vi "Periodic Tasks.vi"(8 "error in":errorcluster) -> ()   [LabVIEW 2016]
doc: "This VI runs in parallel to other tasks. It can contain as many user-defined periodic loops as you need. These can carry out PID or other sorts of timed response."
uses:
  <vilib>/Rock Robotics/WPI/DriverStation/WPI_DriverStationRobotMode2.ctl
  <vilib>/Rock Robotics/Network Tables/NT Write Number.vi
  Robot Global Data.vi
  <vilib>/Rock Robotics/Network Tables/NT Write Boolean.vi
  <vilib>/Rock Robotics/Network Tables/NT Read String.vi
  <vilib>/Rock Robotics/Network Tables/NT Write String.vi
  <vilib>/Rock Robotics/Network Tables/NT Read Number.vi
  <vilib>/Rock Robotics/WPI/Utilities/WPI_GetSetVariantRefNum.vi
  <vilib>/Rock Robotics/Network Tables/NT Read Boolean.vi
  <vilib>/Rock Robotics/Network Tables/NT Write Numeric Array.vi
  <vilib>/Rock Robotics/Network Tables/NT Read Numeric Array.vi
panel:
  out "Shooter Speed":dbl=-0.0
  out "Shooter Encoder 2":dbl(graph)
  out "Shooter Encoder":dbl(graph)
  in  "Voltage Correction Factor":dbl=0.9725 format="%#_13g"
  in  "Ball Detection Fast Time (ms)":u32=20
  out "Channel 1 (Climb Motor)":dbl(graph)
  out "Channel 0 (Climb Motor)":dbl(graph)
  in  "Range":dbl=100.0 format="%#_13g"
  out "Averaged Values":dbl(graph)=25.833333333333332
  out "<5?":i16(graph)=1
  out "Image Width":dbl(graph)=26.0
  in  "Past array Width":dbl[](array[numeric])=[26.0, 26.0, 26.0, 25.0, 26.0, 26.0]
  out "Gear Orient":bool
  out "Gear In":bool
  out "1 Width":dbl=17.0
  out "1 X Axis":dbl=26.0
  out "2 Width":dbl=8.5
  out "2 X Axis":dbl=13.0
  in  "Past array":dbl[](array[numeric])=[-10.0, -10.0, -10.0]
  in  "Lcal Pixy Out":dbl=-10.0
  # "Pixy Code V1 Variables\n      Only here for legacy support if V2 fails.\n\nPixy Code V2 varables are located in\n      \"Pixy Logic Core.vi\""
  # "Factor is 0.9725\nFor voltage 12.8"
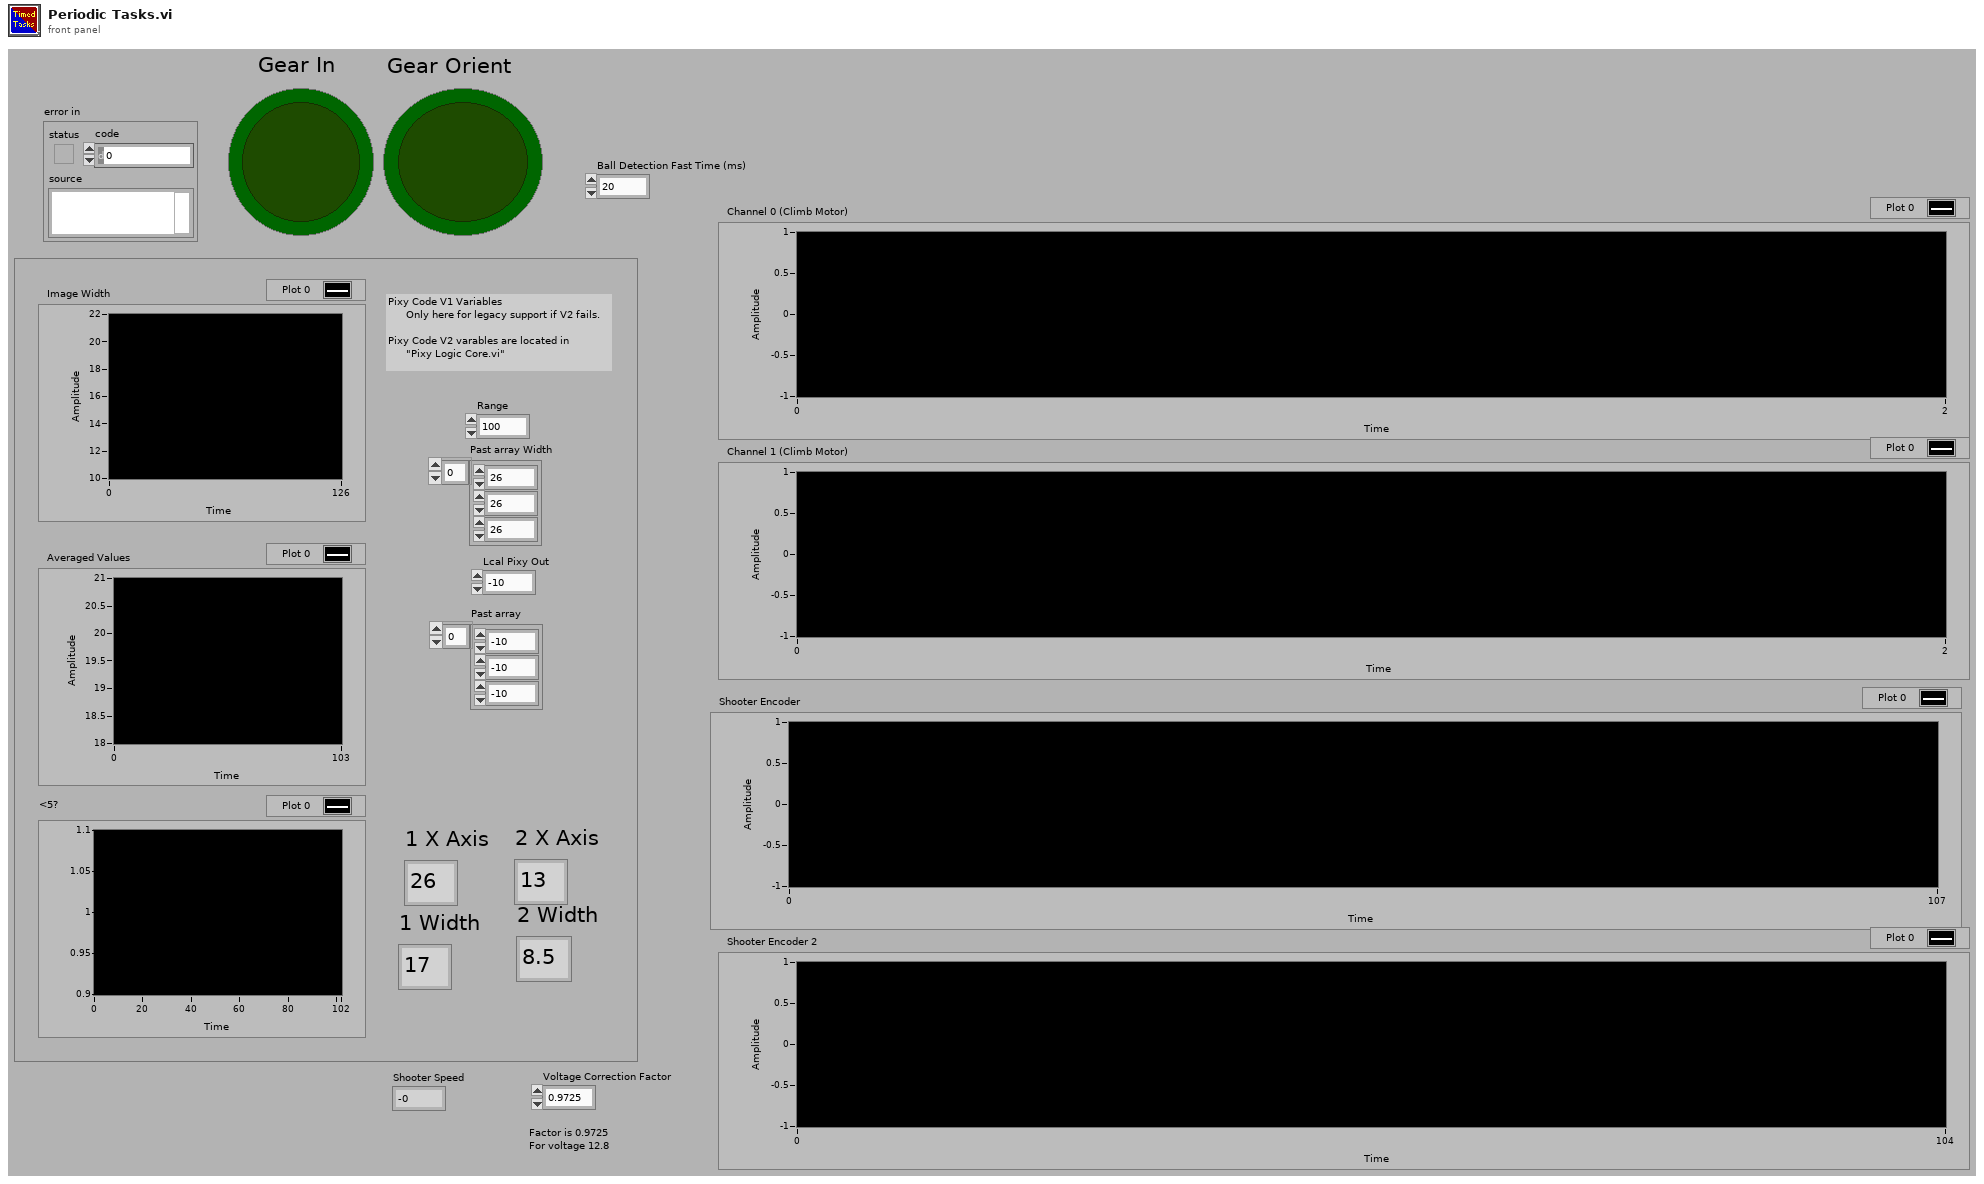
[diagram p1: front panel]
types:
  T1 = typedef "WPI_EncoderDevRef.ctl" = cluster{"DevStatus":errorcluster, "EncoderIndex":T2, "CounterIndex":T3, "DistancePerCount":dbl, "Decoding Type":T4}
  T2 = typedef "FPGA_EncoderIdx.ctl" = enum8{"Enc 0", "Enc 1", "Enc 2", "Enc 3", "Enc 4", "Enc 5", "Enc 6", "Enc 7", "Invalid"}
  T3 = typedef "FPGA_CounterCtrSystemIndex.ctl" = enum8{"Ctr 0", "Ctr 1", "Ctr 2", "Ctr 3", "Ctr 4", "Ctr 5", "Ctr 6", "Ctr 7", "Invalid"}
  T4 = typedef "WPI_EncoderType.ctl" = enum16{"1x", "2x", "4x"}
  T5 = typedef "WPI_SwitchDevRef.ctl" = cluster{"DevStatus":errorcluster, "DIO Channel":T6, "CntIndex":T3, "Normally Closed":bool}
  T6 = typedef "FPGA_DIOChannel.ctl" = enum8{"DIO 0", "DIO 1", "DIO 2", "DIO 3", "DIO 4", "DIO 5", "DIO 6", "DIO 7", "DIO 8", "DIO 9", "DIO MXP 0", "DIO MXP 1", "DIO MXP 2", "DIO MXP 3", "DIO MXP 4", "DIO MXP 5", "DIO MXP 6", "DIO MXP 7", "DIO MXP 8", "DIO MXP 9", "DIO MXP 10", "DIO MXP 11", "DIO MXP 12", "DIO MXP 13", "DIO MXP 14", "DIO MXP 15", "SPI Port CS1", "SPI Port CS2", "SPI Port CS3", "SPI Port MISO", "SPI Port MOSI", "Invalid"}
  T7 = typedef "WPI_ServoDeviceRef.ctl" = cluster{"DeviceStatus":errorcluster, "PWM Channel":T8, "DeadBand":T9}
  T8 = typedef "FPGA_DIOPWMChannel.ctl" = enum8{"PWM 0", "PWM 1", "PWM 2", "PWM 3", "PWM 4", "PWM 5", "PWM 6", "PWM 7", "PWM 8", "PWM 9", "PWM MXP 0", "PWM MXP 1", "PWM MXP 2", "PWM MXP 3", "PWM MXP 4", "PWM MXP 5", "PWM MXP 6", "PWM MXP 7", "PWM MXP 8", "PWM MXP 9", "Invalid"}
  T9 = typedef "WPI_PWMDeadband.ctl" = cluster{"Name":string, "maxPositivePwm":i32, "minPositivePwm":i32, "centerPwm":i32, "maxNegativePwm":i32, "minNegativePwm":i32, "angularRange":u16}
  T10 = typedef "WPI_JoystickDevRef.ctl" = cluster{"Device":T11}
  T11 = typedef "WPI_JoystickDeviceEnum.ctl" = enum16{"USB 0", "USB 1", "USB 2", "USB 3", "USB 4", "USB 5"}
  T12 = typedef "WPI_DriverStationRobotMode2.ctl" = enum16{"Autonomous Disabled", "Autonomous Enabled", "Teleop Disabled", "Teleop Enabled", "Disconnected", "Finish", "Test Disabled", "Test Enabled", "Emergency Stopped"}
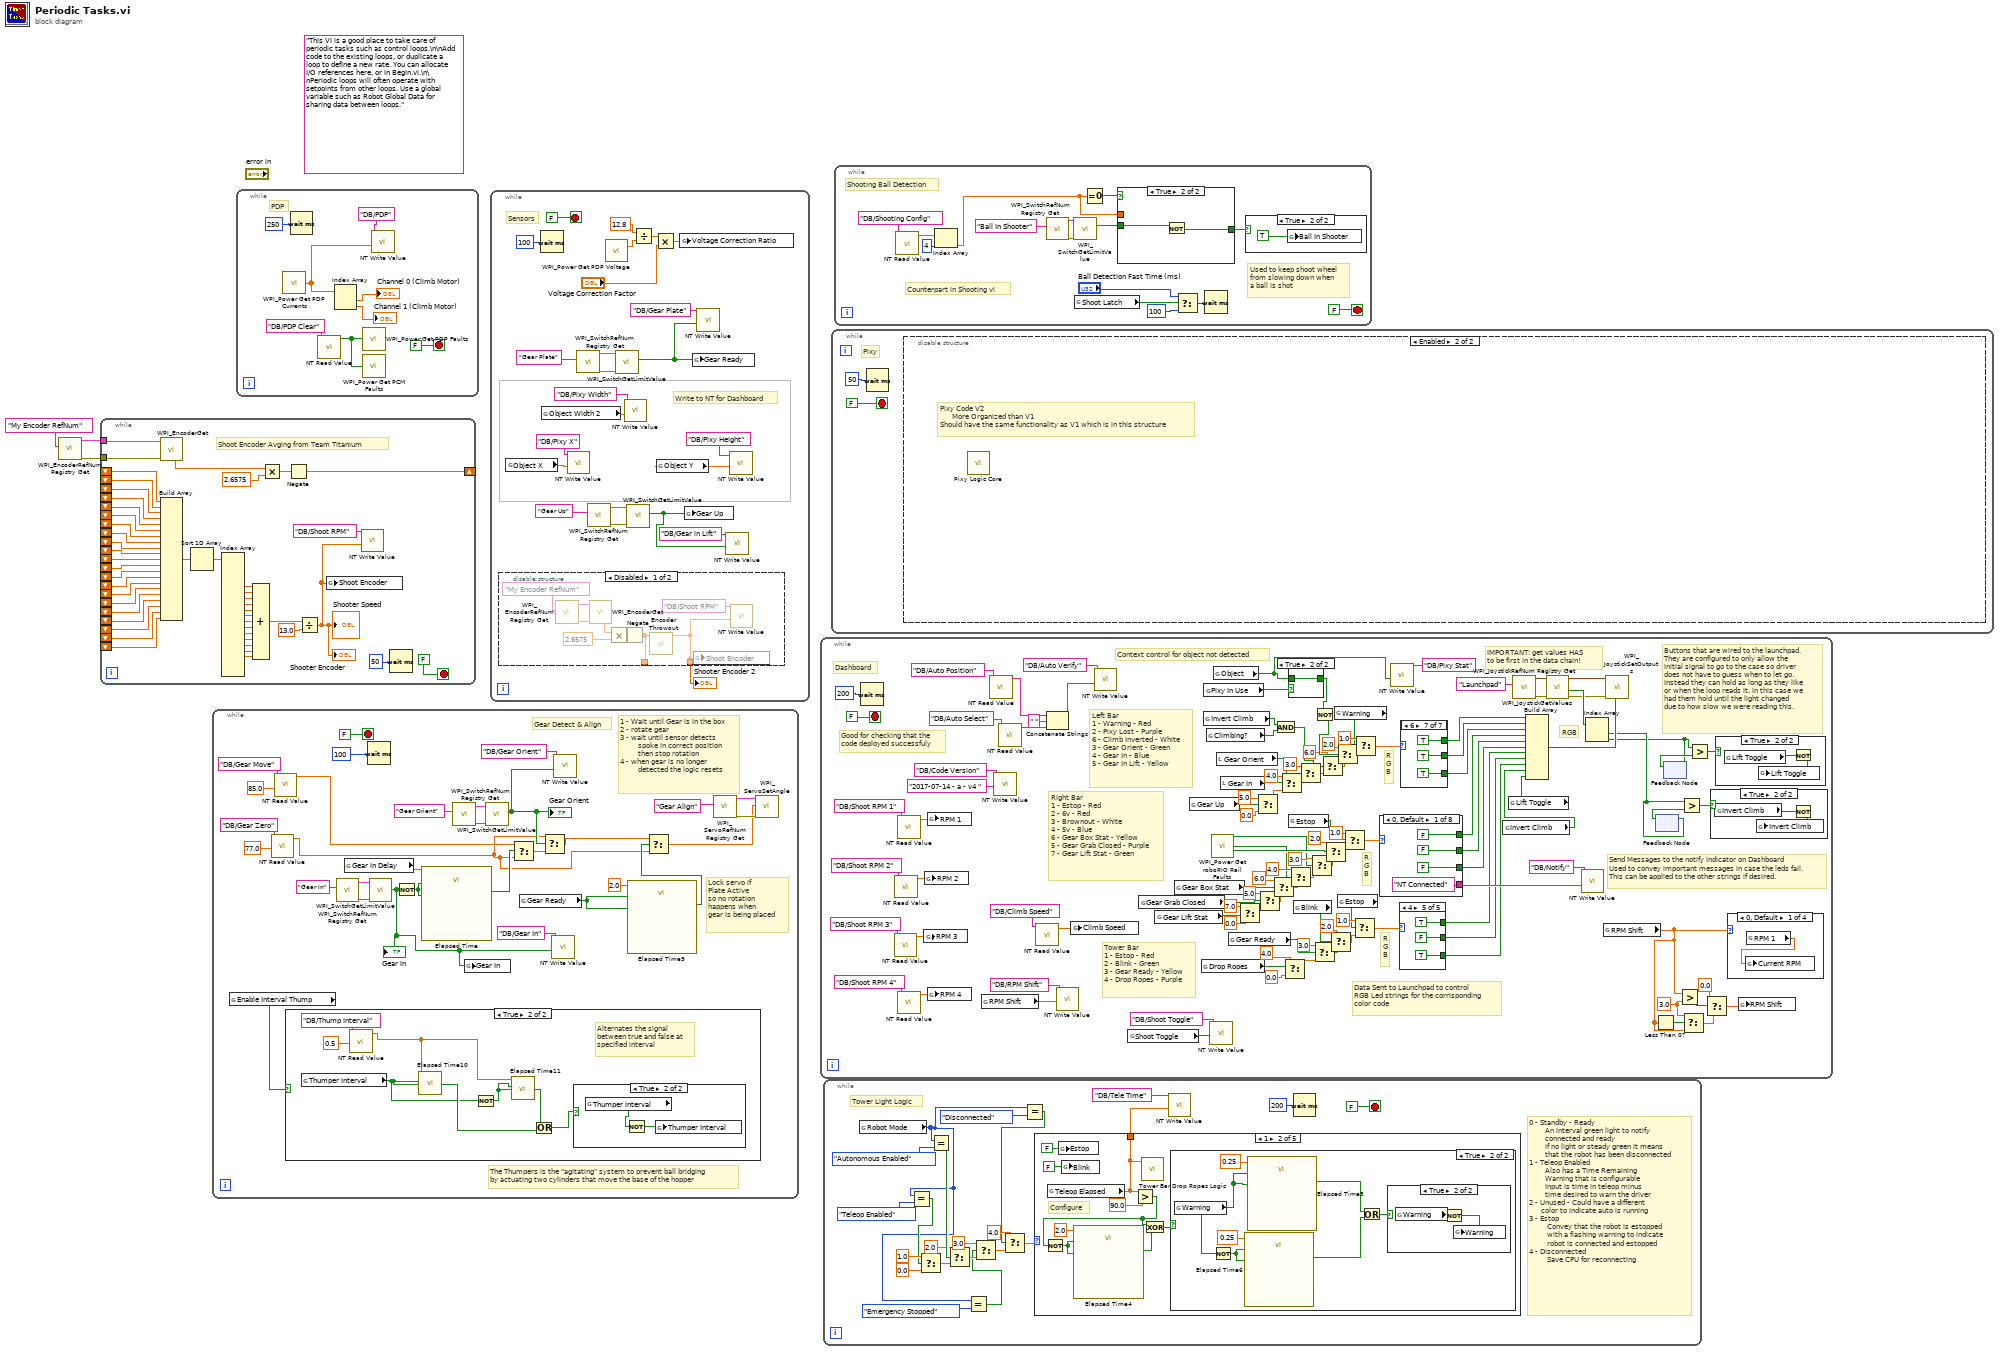
[diagram p0: block diagram]
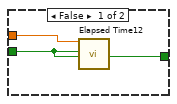
[diagram p2: hidden frame]
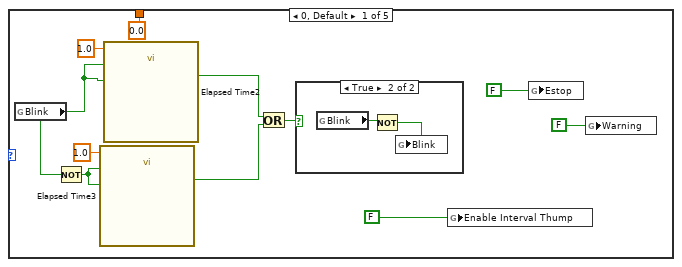
[diagram p4: hidden frame]
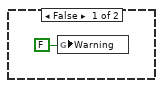
[diagram p6: hidden frame]
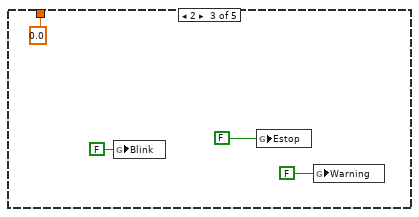
[diagram p8: hidden frame]
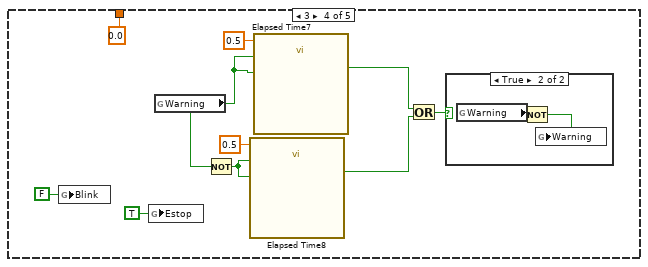
[diagram p9: hidden frame]
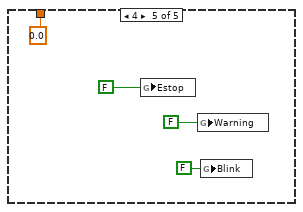
[diagram p11: hidden frame]
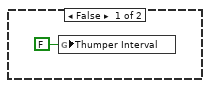
[diagram p12: hidden frame]
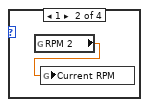
[diagram p14: hidden frame]
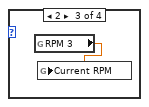
[diagram p15: hidden frame]
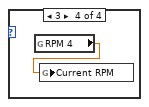
[diagram p16: hidden frame]
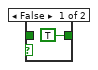
[diagram p19: hidden frame]
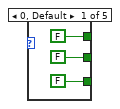
[diagram p20: hidden frame]
diagram:
  (unwired) "This VI is a good place to take care of periodic tasks such as control loops.\n\nAdd code to the existing loops, or duplicate a loop to define a new rate. You can allocate I/O references here, or in Begin.vi.\n\nPeriodic loops will often operate with setpoints from other loops. Use a global variable such as Robot Global Data for sharing data between loops."
  n1 = call <vilib>:"WPI_EncoderRefNum Registry Get.vi"("refnum name"="My Encoder RefNum") -> ("error out"=w1:errorcluster, "EncoderDevRef"=w2:T1)  [unwired: 9 in]
  n2 = while {
    tunnel: w2 -> [w49]
    shift-right: [w46] -> _
    shift-left: _ -> [w45]
    shift-left: _ -> [w44]
    shift-left: _ -> [w43]
    shift-left: _ -> [w42]
    shift-left: _ -> [w41]
    shift-left: _ -> [w40]
    shift-left: _ -> [w39]
    shift-left: _ -> [w38]
    shift-left: _ -> [w37]
    shift-left: _ -> [w36]
    shift-left: _ -> [w35]
    shift-left: _ -> [w34]
    shift-left: _ -> [w33]
    shift-left: _ -> [w32]
    shift-left: _ -> [w31]
    shift-left: _ -> [w30]
    shift-left: _ -> [w17]
    shift-left: _ -> [w16]
    shift-left: _ -> [w15]
    shift-left: _ -> [w14]
    shift-left: _ -> [w13]
    tunnel: w1 -> [w4]
    stop <- FALSE stop-if-true
    # "Shoot Encoder Avging from Team Titanium"
    n3 = call <vilib>:"WPI_EncoderGet.vi"("error in (no error)"=w4, "EncoderDevRef"=w49) -> ("Rate"=w7:dbl)  [unwired: 4 in, 5 out]
    n4 = Build Array(w45, w44, w43, w42, w41, w40, w39, w38, w37, w36, w35, w34, w33, w32, w31, w30, w17, w16, w15, w14, w13) -> (w29:dbl[])
    n5 = Sort 1D Array(array=w29) -> (sorted array=w28:dbl[])
    n6 = Index Array(array=w28) -> (element #4=w27:dbl, element #5=w26:dbl, element #6=w25:dbl, element #7=w24:dbl, element #8=w23:dbl, element #9=w22:dbl, element #10=w21:dbl, element #11=w20:dbl, element #12=w19:dbl, element #13=w18:dbl, element #14=w12:dbl, element #15=w11:dbl, element #16=w10:dbl)  [unwired: 19 in, 6 out]
    n7 = Compound Arithmetic op=ADD(w27, w26, w25, w24, w23, w22, w21, w20, w19, w18, w12, w11, w10) -> (w48:dbl)
    n8 = Multiply(x=w7, y=2.6575 ("x")) -> (x*y=w8:dbl)
    n9 = Negate(x=w8) -> (-x=w46:dbl)
    n10 = Divide(x=w48, y=13.0) -> (x/y=w5:dbl)
    "Shooter Speed" <- w5
    "Shooter Encoder" <- w5
    n11 = global write "Robot Global Data.vi" "Shoot Encoder"(w5) -> ()
    n12 = call-poly <vilib>:"NT Write Value.vi"("Numeric"=w5, "Name"="DB/Shoot RPM") -> ()  [unwired: 9 in, 1 out]
    n13 = Wait (ms)(milliseconds to wait=u32 50) -> ()  [unwired: 1 out]
  }
  n14 = while {
    stop <- FALSE stop-if-true
    # "1 - Wait until Gear is in the box\n2 - rotate gear \n3 - wait until sensor detects \n         spoke in correct position\n         then stop rotation\n4 - when gear is no longer \n         detected the logic resets"
    # "The Thumpers is the \"agitating\" system to prevent ball bridging \nby actuating two cylinders that move the base of the hopper"
    # "Lock servo if\nPlate Active\nso no rotation\nhappens when\ngear is being placed"
    # "Gear Detect & Align"
    n15 = global read "Robot Global Data.vi" "Enable Interval Thump"() -> (w52:bool)
    n16 = call-poly <vilib>:"NT Read Value.vi"("Default Value"=77.0, "Name"="DB/Gear Zero") -> ("Numeric"=w54:dbl)  [unwired: 8 in, 1 out]
    n17 = call-poly <vilib>:"NT Read Value.vi"("Default Value"=85.0, "Name"="DB/Gear Move") -> ("Numeric"=w62:dbl)  [unwired: 8 in, 1 out]
    n18 = case shown="True" w52 {
      frame False {
        n19 = global write "Robot Global Data.vi" "Thumper Interval"(FALSE ("Thumper Interval")) -> ()
      }
      frame True {
        # "Alternates the signal\nbetween true and false at\nspecified interval"
        n20 = global read "Robot Global Data.vi" "Thumper Interval"() -> (w87:bool)
        n21 = call-poly <vilib>:"NT Read Value.vi"("Default Value"=0.5, "Name"="DB/Thump Interval") -> ("Numeric"=w84:dbl)  [unwired: 8 in, 1 out]
        n22 = call "Elapsed Time10"("Time Target (s)"=w84, "Reset"=w87, "Auto Reset"=w87) -> ("Time has Elapsed"=w89:bool)  [unwired: 9 in, 7 out]
        n23 = Not(x=w87) -> (.not. x?=w91:bool)
        n24 = call "Elapsed Time11"("Time Target (s)"=w84, "Reset"=w91, "Auto Reset"=w91) -> ("Time has Elapsed"=w90:bool)  [unwired: 9 in, 7 out]
        n25 = Or(x=w90, y=w89) -> (x .or. y?=w88:bool)
        n26 = case shown="True" w88 {
          frame False {
          }
          frame True {
            n27 = global read "Robot Global Data.vi" "Thumper Interval"() -> (w93:bool)
            n28 = Not(x=w93) -> (.not. x?=w92:bool)
            n29 = global write "Robot Global Data.vi" "Thumper Interval"(w92) -> ()
          }
        }
      }
    }
    n30 = call <vilib>:"WPI_SwitchRefNum Registry Get.vi"("refnum name"="Gear In") -> ("error out"=w79:errorcluster, "SwitchDevRef"=w80:T5)  [unwired: 9 in]
    n31 = global read "Robot Global Data.vi" "Gear In Delay"() -> (w72:dbl)
    n32 = Wait (ms)(milliseconds to wait=u32 100) -> ()  [unwired: 1 out]
    n33 = call <vilib>:"WPI_SwitchGetLimitValue.vi"("error in (no error)"=w79, "SwitchDevRef"=w80) -> ("Switch Pressed"=w53:bool)  [unwired: 7 in, 2 out]
    "Gear In" <- w53
    n34 = Not(x=w53) -> (.not. x?=w73:bool)
    n35 = call "Elapsed Time"("Time Target (s)"=w72, "Reset"=w73, "Auto Reset"=w73) -> ("Time has Elapsed"=w67:bool)  [unwired: 9 in, 7 out]
    n36 = call <vilib>:"WPI_SwitchRefNum Registry Get.vi"("refnum name"="Gear Orient") -> ("error out"=w75:errorcluster, "SwitchDevRef"=w76:T5)  [unwired: 9 in]
    n37 = global write "Robot Global Data.vi" "Gear In"(w53) -> ()
    n38 = call <vilib>:"WPI_SwitchGetLimitValue.vi"("error in (no error)"=w75, "SwitchDevRef"=w76) -> ("Switch Pressed"=w65:bool)  [unwired: 7 in, 2 out]
    "Gear Orient" <- w65
    n39 = Select(t=w62, s=w67, f=w54) -> (s? t:f=w77:dbl)
    n40 = global read "Robot Global Data.vi" "Gear Ready"() -> (w58:bool)
    n41 = Select(t=w54, s=w65, f=w77) -> (s? t:f=w55:dbl)
    n42 = call-poly <vilib>:"NT Write Value.vi"("Boolean"=w53, "Name"="DB/Gear In") -> ()  [unwired: 9 in, 1 out]
    n43 = call-poly <vilib>:"NT Write Value.vi"("Boolean"=w65, "Name"="DB/Gear Orient") -> ()  [unwired: 9 in, 1 out]
    n44 = call "Elapsed Time9"("Time Target (s)"=2.0, "Reset"=w58, "Auto Reset"=w58) -> ("Time has Elapsed"=w56:bool)  [unwired: 9 in, 7 out]
    n45 = Select(t=w55, s=w56, f=w54) -> (s? t:f=w59:dbl)
    n46 = call <vilib>:"WPI_ServoRefNum Registry Get.vi"("refnum name"="Gear Align") -> ("error out"=w68:errorcluster, "ServoDeviceRef"=w69:T7)  [unwired: 9 in]
    n47 = call <vilib>:"WPI_ServoSetAngle.vi"("error in (no error)"=w68, "Angle"=w59, "ServoDeviceRef"=w69) -> ()  [unwired: 7 in, 2 out]
  }
  n48 = while {
    stop <- FALSE stop-if-true
    # "PDP"
    n49 = call <vilib>:"WPI_Power Get PDP Currents.vi"() -> ("all currents (A)"=w96:dbl[])  [unwired: 13 in, 2 out]
    n50 = Wait (ms)(milliseconds to wait=u32 250) -> ()  [unwired: 1 out]
    n51 = call-poly <vilib>:"NT Read Value.vi"("Name"="DB/PDP Clear") -> ("Boolean"=w97:bool)  [unwired: 9 in, 1 out]
    n52 = Index Array(array=w96) -> (element #1=→"Channel 0 (Climb Motor)":dbl, element #2=→"Channel 1 (Climb Motor)":dbl)  [unwired: 2 in]
    n53 = call <vilib>:"WPI_Power Get PDP Faults.vi"("Clear Sticky Faults"=w97) -> ()  [unwired: 10 in, 5 out]
    n54 = call <vilib>:"WPI_Power Get PCM Faults.vi"("Clear Sticky Faults"=w97) -> ()  [unwired: 11 in, 4 out]
    n55 = call-poly <vilib>:"NT Write Value.vi"("Numeric Array"=w96, "Name"="DB/PDP") -> ()  [unwired: 9 in, 1 out]
  }
  n56 = while {
    stop <- FALSE stop-if-true
    # "Write to NT for Dashboard"
    # "Sensors"
    n57 = disable-structure shown="Disabled" {
      disable-tunnel: [w127 _] -> _
      disable-tunnel: [w126 _] -> w102
      frame Disabled {
        n58 = call <vilib>:"WPI_EncoderRefNum Registry Get.vi"("refnum name"="My Encoder RefNum") -> ("error out"=w132:errorcluster, "EncoderDevRef"=w131:T1)  [unwired: 9 in]
        n59 = call <vilib>:"WPI_EncoderGet.vi"("error in (no error)"=w132, "EncoderDevRef"=w131) -> ("Rate"=w130:dbl)  [unwired: 4 in, 5 out]
        n60 = Multiply(x=w130, y=2.6575 ("x")) -> (x*y=w128:dbl)
        n61 = Negate(x=w128) -> (-x=w127:dbl)
        n62 = call "Encoder Throwout.vi"("Input"=w127) -> ("Output"=w126:dbl)  [unwired: 10 in]
        n63 = global write "Robot Global Data.vi" "Shoot Encoder"(w126) -> ()
        n64 = call-poly <vilib>:"NT Write Value.vi"("Numeric"=w126, "Name"="DB/Shoot RPM") -> ()  [unwired: 9 in, 1 out]
      }
      frame Enabled {
      }
    }
    "Shooter Encoder 2" <- w102
    n65 = global read "Robot Global Data.vi" "Object X"() -> (w113:dbl)
    n66 = Wait (ms)(milliseconds to wait=u32 100) -> ()  [unwired: 1 out]
    n67 = global read "Robot Global Data.vi" "Object Width 2"() -> (w115:dbl)
    n68 = call-poly <vilib>:"NT Write Value.vi"("Numeric"=w113, "Name"="DB/Pixy X") -> ()  [unwired: 9 in, 1 out]
    n69 = call <vilib>:"WPI_SwitchRefNum Registry Get.vi"("refnum name"="Gear Plate") -> ("error out"=w123:errorcluster, "SwitchDevRef"=w122:T5)  [unwired: 9 in]
    n70 = call <vilib>:"WPI_SwitchRefNum Registry Get.vi"("refnum name"="Gear Up") -> ("error out"=w112:errorcluster, "SwitchDevRef"=w111:T5)  [unwired: 9 in]
    n71 = call <vilib>:"WPI_Power Get PDP Voltage.vi"() -> ("voltage (V)"=w106:dbl)  [unwired: 14 in, 1 out]
    n72 = call <vilib>:"WPI_SwitchGetLimitValue.vi"("error in (no error)"=w123, "SwitchDevRef"=w122) -> ("Switch Pressed"=w119:bool)  [unwired: 7 in, 2 out]
    n73 = call-poly <vilib>:"NT Write Value.vi"("Numeric"=w115, "Name"="DB/Pixy Width") -> ()  [unwired: 9 in, 1 out]
    n74 = call <vilib>:"WPI_SwitchGetLimitValue.vi"("error in (no error)"=w112, "SwitchDevRef"=w111) -> ("Switch Pressed"=w108:bool)  [unwired: 7 in, 2 out]
    n75 = Divide(x=12.8, y=w106) -> (x/y=w105:dbl)
    n76 = Multiply(x=w105, y="Voltage Correction Factor") -> (x*y=w103:dbl)
    n77 = global read "Robot Global Data.vi" "Object Y"() -> (w114:dbl)
    n78 = global write "Robot Global Data.vi" "Voltage Correction Ratio"(w103) -> ()
    n79 = global write "Robot Global Data.vi" "Gear Up"(w108) -> ()
    n80 = global write "Robot Global Data.vi" "Gear Ready"(w119) -> ()
    n81 = call-poly <vilib>:"NT Write Value.vi"("Boolean"=w119, "Name"="DB/Gear Plate") -> ()  [unwired: 9 in, 1 out]
    n82 = call-poly <vilib>:"NT Write Value.vi"("Boolean"=w108, "Name"="DB/Gear in Lift") -> ()  [unwired: 9 in, 1 out]
    n83 = call-poly <vilib>:"NT Write Value.vi"("Numeric"=w114, "Name"="DB/Pixy Height") -> ()  [unwired: 9 in, 1 out]
  }
  n84 = while {
    stop <- FALSE stop-if-true
    w162 = 3.0 ("y")
    # "Good for checking that the\ncode deployed successfuly"
    # "IMPORTANT: get values HAS \nto be first in the data chain!"
    # "Buttons that are wired to the launchpad.\nThey are configured to only allow the \ninitial signal to go to the case so driver\ndoes not have to guess when to let go.\nInstead they can hold as long as they like\nor when the loop reads it. In this case we\nhad them hold until the light changed \ndue to how slow we were reading this."
    # "Context control for object not detected"
    # "Send Messages to the notify indicator on Dashboard\nUsed to convey important messages in case the leds fail.\nThis can be applied to the other strings if desired."
    # "R\nG\nB"
    # "R\nG\nB"
    # "R\nG\nB"
    # "Data Sent to Launchpad to control\nRGB Led strings for the corrisponding \ncolor code"
    # "Left Bar\n1 - Warning - Red\n2 - Pixy Lost - Purple \n6 - Climb Inverted - White\n3 - Gear Orient - Green\n4 - Gear In - Blue\n5 - Gear In Lift - Yellow"
    # "RGB"
    # "Tower Bar\n1 - Estop - Red\n2 - Blink - Green\n3 - Gear Ready - Yellow\n4 - Drop Ropes - Purple"
    # "Right Bar\n1 - Estop - Red\n2 - 6v - Red\n3 - Brownout - White\n4 - 5v - Blue\n6 - Gear Box Stat - Yellow\n5 - Gear Grab Closed - Purple\n7 - Gear Lift Stat - Green"
    # "Dashboard"
    n85 = Wait (ms)(milliseconds to wait=u32 200) -> ()  [unwired: 1 out]
    n86 = call-poly <vilib>:"NT Read Value.vi"("Name"="DB/Shoot RPM 3") -> ("Numeric"=w233:dbl)  [unwired: 9 in, 1 out]
    n87 = call-poly <vilib>:"NT Read Value.vi"("Name"="DB/Shoot RPM 2") -> ("Numeric"=w235:dbl)  [unwired: 9 in, 1 out]
    n88 = call-poly <vilib>:"NT Read Value.vi"("Name"="DB/Shoot RPM 1") -> ("Numeric"=w239:dbl)  [unwired: 9 in, 1 out]
    n89 = call-poly <vilib>:"NT Read Value.vi"("Name"="DB/Shoot RPM 4") -> ("Numeric"=w231:dbl)  [unwired: 9 in, 1 out]
    n90 = global write "Robot Global Data.vi" "RPM 3"(w233) -> ()
    n91 = global write "Robot Global Data.vi" "RPM 2"(w235) -> ()
    n92 = global write "Robot Global Data.vi" "RPM 1"(w239) -> ()
    n93 = global write "Robot Global Data.vi" "RPM 4"(w231) -> ()
    n94 = global read "Robot Global Data.vi" "RPM Shift"() -> (w229:dbl)
    n95 = call-poly <vilib>:"NT Read Value.vi"("Name"="DB/Auto Position") -> ("String"=w249:string)  [unwired: 9 in, 1 out]
    n96 = call-poly <vilib>:"NT Write Value.vi"("String"="2017-07-14 - a - v4 ", "Name"="DB/Code Version") -> ()  [unwired: 9 in, 1 out]
    n97 = call-poly <vilib>:"NT Read Value.vi"("Name"="DB/Auto Select") -> ("String"=w250:string)  [unwired: 9 in, 1 out]
    n98 = call-poly <vilib>:"NT Read Value.vi"("Name"="DB/Climb Speed") -> ("Numeric"=w237:dbl)  [unwired: 9 in, 1 out]
    n99 = Concatenate Strings(w249, " " ("string"), w250) -> (w248:string)
    n100 = call-poly <vilib>:"NT Write Value.vi"("Numeric"=w229, "Name"="DB/RPM Shift") -> ()  [unwired: 9 in, 1 out]
    n101 = global write "Robot Global Data.vi" "Climb Speed"(w237) -> ()
    n102 = call-poly <vilib>:"NT Write Value.vi"("String"=w248, "Name"="DB/Auto Verify") -> ()  [unwired: 9 in, 1 out]
    n103 = global read "Robot Global Data.vi" "Shoot Toggle"() -> (w150:bool)
    n104 = global read "Robot Global Data.vi" "Gear Grab Closed"() -> (w143:bool)
    n105 = global read "Robot Global Data.vi" "Gear Lift Stat"() -> (w152:bool)
    n106 = global read "Robot Global Data.vi" "Gear Box Stat"() -> (w144:bool)
    n107 = global read "Robot Global Data.vi" "Gear Up"() -> (w147:bool)
    n108 = global read "Robot Global Data.vi" "Drop Ropes"() -> (w135:bool)
    n109 = global read "Robot Global Data.vi" "Invert Climb"() -> (w138:bool)
    n110 = global read "Robot Global Data.vi" "Pixy In Use"() -> (w180:bool)
    n111 = global read "Robot Global Data.vi" "Climbing?"() -> (w137:bool)
    n112 = call-poly <vilib>:"NT Write Value.vi"("Boolean"=w150, "Name"="DB/Shoot Toggle") -> ()  [unwired: 9 in, 1 out]
    n113 = call <vilib>:"WPI_Power Get roboRIO Rail Faults.vi"() -> ("Input Voltage Brown Out"=w203:bool, "5 V User Rail Short"=w204:bool, "6 V User Rail Short"=w205:bool)  [unwired: 10 in, 3 out]
    n114 = global read "Robot Global Data.vi" "Object"() -> (w174:bool)
    n115 = local read "Gear Orient"() -> (w182:bool)
    n116 = local read "Gear In"() -> (w181:bool)
    n117 = global read "Robot Global Data.vi" "Gear Ready"() -> (w184:bool)
    n118 = Select(t=7.0, s=w152, f=0.0) -> (s? t:f=w155:dbl)
    n119 = Select(t=5.0, s=w147, f=0.0) -> (s? t:f=w148:dbl)
    n120 = Select(t=5.0, s=w143, f=w155) -> (s? t:f=w206:dbl)
    n121 = Select(t=6.0, s=w144, f=w206) -> (s? t:f=w207:dbl)
    n122 = And(x=w138, y=w137) -> (x .and. y?=w136:bool)
    n123 = Select(t=4.0, s=w181, f=w148) -> (s? t:f=w222:dbl)
    n124 = Select(t=4.0, s=w135, f=0.0) -> (s? t:f=w192:dbl)
    n125 = case shown="True" w180 {
      tunnel: [TRUE ("Object") w262] -> w178
      tunnel: w174 -> [_ w262]
      frame False {
      }
      frame True {
      }
    }
    n126 = global read "Robot Global Data.vi" "Estop"() -> (w209:bool)
    n127 = Select(t=4.0, s=w204, f=w207) -> (s? t:f=w214:dbl)
    n128 = global read "Robot Global Data.vi" "Blink"() -> (w185:bool)
    n129 = Select(t=3.0, s=w182, f=w222) -> (s? t:f=w139:dbl)
    n130 = Select(t=3.0, s=w203, f=w214) -> (s? t:f=w215:dbl)
    n131 = Select(t=3.0, s=w184, f=w192) -> (s? t:f=w193:dbl)
    n132 = Not(x=w178) -> (.not. x?=w179:bool)
    n133 = Select(t=6.0, s=w136, f=w139) -> (s? t:f=w141:dbl)
    n134 = Select(t=2.0, s=w205, f=w215) -> (s? t:f=w216:dbl)
    n135 = Select(t=2.0, s=w185, f=w193) -> (s? t:f=w194:dbl)
    n136 = global read "Robot Global Data.vi" "Warning"() -> (w196:bool)
    n137 = Select(t=2.0, s=w179, f=w141) -> (s? t:f=w226:dbl)
    n138 = global read "Robot Global Data.vi" "Estop"() -> (w186:bool)
    n139 = Select(t=1.0, s=w209, f=w216) -> (s? t:f=w210:dbl)
    n140 = Select(t=1.0, s=w186, f=w194) -> (s? t:f=w195:dbl)
    n141 = Select(t=1.0, s=w196, f=w226) -> (s? t:f=w227:dbl)
    n142 = case shown="0, Default" w210 {
      tunnel: [FALSE TRUE TRUE TRUE FALSE TRUE TRUE FALSE] -> w199
      tunnel: [FALSE FALSE FALSE TRUE FALSE FALSE TRUE TRUE] -> w198
      tunnel: [FALSE FALSE FALSE TRUE TRUE TRUE FALSE FALSE] -> w197
      tunnel: ["NT Connected" ("String") "EStop - Reset Rio" ("String") "6v Rail Short" ("String") "Brownout" ("String") "5v Rail Short" ("String") "NT Connected" ("String") "NT Connected" ("String") "NT Connected" ("String")] -> w217
      frame 0, Default {
      }
      frame 1 {
      }
      frame 2 {
      }
      frame 3 {
      }
      frame 4 {
      }
      frame 5 {
      }
      frame 6 {
      }
      frame 7 {
      }
    }
    n143 = call-poly <vilib>:"NT Write Value.vi"("Boolean"=w174, "Name"="DB/Pixy Stat") -> ()  [unwired: 9 in, 1 out]
    n144 = case shown="4" w195 {
      tunnel: [FALSE TRUE FALSE TRUE TRUE] -> w177
      tunnel: [FALSE FALSE TRUE TRUE FALSE] -> w176
      tunnel: [FALSE FALSE FALSE FALSE TRUE] -> w175
      frame 0, Default {
      }
      frame 1 {
      }
      frame 2 {
      }
      frame 3 {
      }
      frame 4 {
      }
    }
    n145 = case shown="6" w227 {
      tunnel: [FALSE TRUE TRUE FALSE FALSE TRUE TRUE] -> w225
      tunnel: [FALSE FALSE FALSE TRUE FALSE TRUE TRUE] -> w224
      tunnel: [FALSE FALSE TRUE FALSE TRUE FALSE TRUE] -> w223
      frame 0, Default {
      }
      frame 1 {
      }
      frame 2 {
      }
      frame 3 {
      }
      frame 4 {
      }
      frame 5 {
      }
      frame 6 {
      }
    }
    n146 = global read "Robot Global Data.vi" "Invert Climb"() -> (w142:bool)
    n147 = global read "Robot Global Data.vi" "Lift Toggle"() -> (w149:bool)
    n148 = call <vilib>:"WPI_JoystickRefNum Registry Get.vi"("refnum name"="Launchpad") -> ("error out"=w161:errorcluster, "JoystickDevRef"=w160:T10)  [unwired: 9 in]
    n149 = Build Array(w225, w224, w223, w199, w198, w197, w177, w176, w175, w142, w149) -> (w200:bool[])
    n150 = call <vilib>:"WPI_JoystickGetValues.vi"("error in (no error)"=w161, "JoystickDevRef"=w160) -> ("error out"=w158:errorcluster, "Buttons"=w173:bool[], "JoystickDevRef"=w159:T10)  [unwired: 5 in, 2 out]
    n151 = call-poly <vilib>:"NT Write Value.vi"("String"=w217, "Name"="DB/Notify") -> ()  [unwired: 9 in, 1 out]
    n152 = Index Array(array=w173) -> (element #1=w157:bool, element #2=w156:bool)  [unwired: 2 in]
    n153 = global read "Robot Global Data.vi" "RPM Shift"() -> (w163:dbl)
    n154 = call <vilib>:"WPI_JoystickSetOutputs.vi"("Outputs"=w200, "error in (no error)"=w158, "JoystickDevRef"=w159) -> ()  [unwired: 7 in, 2 out]
    n155 = Less Than 0?(x=w163) -> (x < 0?=w166:bool)
    n156 = feedback #1() -> (w169:bool)  [unwired: 1 in]
    n157 = feedback-in #1(w157) -> ()
    n158 = feedback #2() -> (w171:bool)  [unwired: 1 in]
    n159 = feedback-in #2(w156) -> ()
    n160 = Greater?(x=w163, y=w162) -> (0:w165:bool)
    n161 = Greater?(x=w157, y=w169) -> (0:w170:bool)
    n162 = Select(t=w162, s=w166, f=w163) -> (s? t:f=w167:dbl)
    n163 = Greater?(x=w156, y=w171) -> (0:w172:bool)
    n164 = Select(t=0.0, s=w165, f=w167) -> (s? t:f=w168:dbl)
    n165 = case shown="True" w170 {
      frame False {
      }
      frame True {
        n166 = global read "Robot Global Data.vi" "Invert Climb"() -> (w258:bool)
        n167 = Not(x=w258) -> (.not. x?=w257:bool)
        n168 = global write "Robot Global Data.vi" "Invert Climb"(w257) -> ()
      }
    }
    n169 = case shown="True" w172 {
      frame False {
      }
      frame True {
        n170 = global read "Robot Global Data.vi" "Lift Toggle"() -> (w260:bool)
        n171 = Not(x=w260) -> (.not. x?=w259:bool)
        n172 = global write "Robot Global Data.vi" "Lift Toggle"(w259) -> ()
      }
    }
    n173 = case shown="0, Default" w163 {
      frame 0, Default {
        n174 = global read "Robot Global Data.vi" "RPM 1"() -> (w253:dbl)
        n175 = global write "Robot Global Data.vi" "Current RPM"(w253) -> ()
      }
      frame 1 {
        n176 = global read "Robot Global Data.vi" "RPM 2"() -> (w254:dbl)
        n177 = global write "Robot Global Data.vi" "Current RPM"(w254) -> ()
      }
      frame 2 {
        n178 = global read "Robot Global Data.vi" "RPM 3"() -> (w255:dbl)
        n179 = global write "Robot Global Data.vi" "Current RPM"(w255) -> ()
      }
      frame 3 {
        n180 = global read "Robot Global Data.vi" "RPM 4"() -> (w256:dbl)
        n181 = global write "Robot Global Data.vi" "Current RPM"(w256) -> ()
      }
    }
    n182 = global write "Robot Global Data.vi" "RPM Shift"(w168) -> ()
  }
  n183 = while {
    stop <- FALSE stop-if-true
    # "0 - Standby - Ready\n        An interval green light to notify\n        connected and ready\n        if no light or steady green it means\n        that the robot has been disconnected\n1 - Teleop Enabled\n        Also has a Time Remaining\n        Warning that is configurable\n        Input is time in teleop minus \n        time desired to warn the driver\n2 - Unused - Could have a different\n      color to indicate auto is running\n3 - Estop\n         Convey that the robot is estopped\n         with a flashing warning to indicate\n         robot is connected and estopped\n4 - Disconnected\n         Save CPU for reconnecting"
    # "Tower Light Logic"
    n184 = global read "Robot Global Data.vi" "Robot Mode"() -> (w331:T12)
    n185 = Equal?(x=w331, y=WPI_DriverStationRobotMode2."Teleop Enabled") -> (x = y?=w342:bool)
    n186 = Select(t=1.0, s=w342, f=0.0) -> (s? t:f=w348:dbl)
    n187 = Equal?(x=w331, y=WPI_DriverStationRobotMode2."Autonomous Enabled") -> (x = y?=w344:bool)
    n188 = Select(t=2.0, s=w344, f=w348) -> (s? t:f=w341:dbl)
    n189 = Equal?(x=w331, y=WPI_DriverStationRobotMode2."Emergency Stopped") -> (x = y?=w338:bool)
    n190 = Select(t=3.0, s=w338, f=w341) -> (s? t:f=w339:dbl)
    n191 = Equal?(x=w331, y=WPI_DriverStationRobotMode2."Disconnected") -> (x = y?=w335:bool)
    n192 = Select(t=4.0, s=w335, f=w339) -> (s? t:f=w334:dbl)
    n193 = case shown="1" w334 {
      tunnel: [0.0 ("Teleop Elapsed") w366 0.0 ("Teleop Elapsed") 0.0 ("Teleop Elapsed") 0.0 ("Teleop Elapsed")] -> w332
      frame 0, Default {
        n194 = global read "Robot Global Data.vi" "Blink"() -> (w357:bool)
        n195 = Not(x=w357) -> (.not. x?=w358:bool)
        n196 = call "Elapsed Time3"("Time Target (s)"=1.0, "Reset"=w358, "Auto Reset"=w358) -> ("Time has Elapsed"=w359:bool)  [unwired: 9 in, 7 out]
        n197 = call "Elapsed Time2"("Time Target (s)"=1.0, "Reset"=w357, "Auto Reset"=w357) -> ("Time has Elapsed"=w360:bool)  [unwired: 9 in, 7 out]
        n198 = Or(x=w360, y=w359) -> (x .or. y?=w361:bool)
        n199 = case shown="True" w361 {
          frame False {
          }
          frame True {
            n200 = global read "Robot Global Data.vi" "Blink"() -> (w365:bool)
            n201 = Not(x=w365) -> (.not. x?=w364:bool)
            n202 = global write "Robot Global Data.vi" "Blink"(w364) -> ()
          }
        }
        n203 = global write "Robot Global Data.vi" "Enable Interval Thump"(FALSE) -> ()
        n204 = global write "Robot Global Data.vi" "Estop"(FALSE ("Blink")) -> ()
        n205 = global write "Robot Global Data.vi" "Warning"(FALSE ("Blink")) -> ()
      }
      frame 1 {
        # "Configure"
        n206 = global read "Robot Global Data.vi" "Teleop Elapsed"() -> (w366:dbl)
        n207 = global write "Robot Global Data.vi" "Estop"(FALSE ("Blink")) -> ()
        n208 = global write "Robot Global Data.vi" "Blink"(FALSE ("Blink")) -> ()
        n209 = Greater?(x=w366, y=90.0) -> (0:w370:bool)
        n210 = Not(x=w370) -> (.not. x?=w373:bool)
        n211 = call "Elapsed Time4"("Time Target (s)"=2.0, "Reset"=w373, "Auto Reset"=w373) -> ("Time has Elapsed"=w368:bool)  [unwired: 9 in, 7 out]
        n212 = call "Tower Bar Drop Ropes Logic.vi"("Input"=w366) -> ()  [unwired: 11 in]
        n213 = Exclusive Or(1:w368, 2:w370) -> (0:w369:bool)
        n214 = case shown="True" w369 {
          frame False {
            n215 = global write "Robot Global Data.vi" "Warning"(FALSE ("Blink")) -> ()
          }
          frame True {
            n216 = global read "Robot Global Data.vi" "Warning"() -> (w376:bool)
            n217 = Not(x=w376) -> (.not. x?=w377:bool)
            n218 = call "Elapsed Time6"("Time Target (s)"=0.25, "Reset"=w377, "Auto Reset"=w377) -> ("Time has Elapsed"=w378:bool)  [unwired: 9 in, 7 out]
            n219 = call "Elapsed Time5"("Time Target (s)"=0.25, "Reset"=w376, "Auto Reset"=w376) -> ("Time has Elapsed"=w379:bool)  [unwired: 9 in, 7 out]
            n220 = Or(x=w379, y=w378) -> (x .or. y?=w380:bool)
            n221 = case shown="True" w380 {
              frame False {
              }
              frame True {
                n222 = global read "Robot Global Data.vi" "Warning"() -> (w384:bool)
                n223 = Not(x=w384) -> (.not. x?=w383:bool)
                n224 = global write "Robot Global Data.vi" "Warning"(w383) -> ()
              }
            }
          }
        }
      }
      frame 2 {
        n225 = global write "Robot Global Data.vi" "Blink"(FALSE ("Blink")) -> ()
        n226 = global write "Robot Global Data.vi" "Estop"(FALSE ("Blink")) -> ()
        n227 = global write "Robot Global Data.vi" "Warning"(FALSE ("Blink")) -> ()
      }
      frame 3 {
        n228 = global write "Robot Global Data.vi" "Blink"(FALSE ("Blink")) -> ()
        n229 = global write "Robot Global Data.vi" "Estop"(TRUE ("Estop")) -> ()
        n230 = global read "Robot Global Data.vi" "Warning"() -> (w391:bool)
        n231 = Not(x=w391) -> (.not. x?=w393:bool)
        n232 = call "Elapsed Time8"("Time Target (s)"=0.5, "Reset"=w393, "Auto Reset"=w393) -> ("Time has Elapsed"=w394:bool)  [unwired: 9 in, 7 out]
        n233 = call "Elapsed Time7"("Time Target (s)"=0.5, "Reset"=w391, "Auto Reset"=w391) -> ("Time has Elapsed"=w395:bool)  [unwired: 9 in, 7 out]
        n234 = Or(x=w395, y=w394) -> (x .or. y?=w396:bool)
        n235 = case shown="True" w396 {
          frame False {
          }
          frame True {
            n236 = global read "Robot Global Data.vi" "Warning"() -> (w400:bool)
            n237 = Not(x=w400) -> (.not. x?=w399:bool)
            n238 = global write "Robot Global Data.vi" "Warning"(w399) -> ()
          }
        }
      }
      frame 4 {
        n239 = global write "Robot Global Data.vi" "Estop"(FALSE ("Blink")) -> ()
        n240 = global write "Robot Global Data.vi" "Warning"(FALSE ("Blink")) -> ()
        n241 = global write "Robot Global Data.vi" "Blink"(FALSE ("Blink")) -> ()
      }
    }
    n242 = call-poly <vilib>:"NT Write Value.vi"("Numeric"=w332, "Name"="DB/Tele Time") -> ()  [unwired: 9 in, 1 out]
    n243 = Wait (ms)(milliseconds to wait=u32 200) -> ()  [unwired: 1 out]
  }
  n244 = while {
    stop <- FALSE stop-if-true
    # "Pixy"
    n245 = Wait (ms)(milliseconds to wait=u32 50) -> ()  [unwired: 1 out]
    n246 = disable-structure shown="Enabled" {
      frame Disabled {
        # "Pixy Code V1"
        # "Note: More documentation is in the vis used here"
        # "NOTE: Our Pixycam was\nmounted sideways hence,\nthe opposite wiring on\nthe Global Variables"
        # "Keeps Value if pixy is lost"
        # "Cuts off if no object\nis found by pixy"
        # "Select case depending\non whether or not two\nobjects are detected"
        # "Graphs"
        # "Logic to tell if an object was detected by pixy"
        # "Temporary for passthrough testing (Skiping the Object error vi): 160 Original: 0"
        n247 = call "PixyGetFrame.vi"() -> ("Frame"=w415:string)  [unwired: 11 in]
        n248 = call "PixyGetObject.vi"("Input Frame"=w415) -> ("Remainder of Frame"=w414:string, "Object"=w413:string, "Empty?"=w411:bool)  [unwired: 8 in]
        n249 = Not(x=w411) -> (.not. x?=w417:bool)
        n250 = case shown="False" w411 {
          tunnel: [w438 w486] -> w409
          tunnel: w414 -> [w437 _]
          tunnel: w413 -> [w435 _]
          tunnel: [w433 FALSE] -> w412
          tunnel: [w427 w484] -> w408
          frame False {
            # "Used to delay object width averaging by five values to help clear the table\nof the values that were read when moving into position to use this code"
            # "Rejection logic to reduce noise"
            # "Graph to see when a \nvalue was rejected"
            n251 = call "PixyGetObject.vi"("Input Frame"=w437) -> ("Object"=w434:string, "Empty?"=w436:bool)  [unwired: 8 in, 1 out]
            n252 = global read "Robot Global Data.vi" "NumValuesInTable"() -> (w430:dbl)
            n253 = case shown="True" w436 {
              tunnel: [w463 w477] -> w438
              tunnel: w435 -> [w459 w474]
              tunnel: w434 -> [w458 _]
              tunnel: [w455 w473] -> w433
              tunnel: [w445 w470] -> w427
              frame False {
                # "Two objects found"
                # "Average both objects then\ncalculate as normal"
                # "Average Table"
                n254 = call "PixyHexDecode.vi"("Object"=w459) -> ("X"=w444:dbl, "Y"=w447:dbl, "Width"=w450:dbl)  [unwired: 10 in, 2 out]
                n255 = call "PixyHexDecode.vi"("Object"=w458) -> ("X"=w443:dbl, "Y"=w446:dbl, "Width"=w449:dbl)  [unwired: 10 in, 2 out]
                n256 = Add(x=w447, y=w446) -> (x+y=w461:dbl)
                n257 = Divide(x=w461, y=2.0) -> (x/y=w457:dbl)
                n258 = Add(x=w444, y=w443) -> (x+y=w454:dbl)
                n259 = local read "Past array"() -> (w469:dbl[])
                n260 = call "PixyObjectErrorXAxis.vi"("Input Value"=w457) -> ("Output"=w456:dbl, "Object In Parameters"=w455:bool)  [unwired: 9 in]
                n261 = Divide(x=w454, y=2.0) -> (x/y=w445:dbl)
                "2 X Axis" <- w445
                n262 = Add(x=w450, y=w449) -> (x+y=w452:dbl)
                n263 = Index Array(array=w469) -> (element #1=w468:dbl, element #2=w467:dbl)  [unwired: 3 in, 1 out]
                n264 = Divide(x=w452, y=2.0) -> (x/y=w448:dbl)
                "2 Width" <- w448
                n265 = global write "Robot Global Data.vi" "Object Height"(w448) -> ()
                n266 = Add(x=w468, y=w467) -> (x+y=w466:dbl)
                n267 = Build Array(w456, w468, w467) -> (w462:dbl[])
                n268 = local write "Past array"(w462) -> ()
                n269 = Add(x=w466, y=w456) -> (x+y=w465:dbl)
                n270 = Divide(x=w465, y=3.0) -> (x/y=w463:dbl)
              }
              frame True {
                # "One Object found"
                # "Average Table"
                n271 = call "PixyHexDecode.vi"("Object"=w474) -> ("X"=w470:dbl, "Y"=w471:dbl, "Width"=w472:dbl)  [unwired: 10 in, 2 out]
                "1 Width" <- w472
                "1 X Axis" <- w470
                n272 = call "PixyObjectErrorXAxis.vi"("Input Value"=w471) -> ("Output"=w476:dbl, "Object In Parameters"=w473:bool)  [unwired: 9 in]
                n273 = global write "Robot Global Data.vi" "Object Height"(w472) -> ()
                n274 = local read "Past array"() -> (w483:dbl[])
                n275 = Index Array(array=w483) -> (element #1=w482:dbl, element #2=w481:dbl)  [unwired: 3 in, 1 out]
                n276 = Add(x=w482, y=w481) -> (x+y=w480:dbl)
                n277 = Build Array(w476, w482, w481) -> (w475:dbl[])
                n278 = Add(x=w480, y=w476) -> (x+y=w479:dbl)
                n279 = local write "Past array"(w475) -> ()
                n280 = Divide(x=w479, y=3.0) -> (x/y=w477:dbl)
              }
            }
            n281 = Add(x=w430, y=1.0) -> (x+y=w428:dbl)
            n282 = global write "Robot Global Data.vi" "NumValuesInTable"(w428) -> ()
            n283 = global read "Robot Global Data.vi" "Object Width"() -> (w426)
            n284 = global read "Robot Global Data.vi" "NumValuesInTable"() -> (w432:dbl)
            n285 = Add(x=w426, y="Range") -> (x+y=w423:dbl)
            n286 = Subtract(x=w426, y="Range") -> (x-y=w424:dbl)
            n287 = Less?(x=w432, y=5.0) -> (x < y?=w421:bool)
            n288 = In Range and Coerce(upper limit=w423, x=w427, lower limit=w424) -> (In Range?=w422:bool)  [unwired: 1 out]
            n289 = Or(x=w422, y=w421) -> (x .or. y?=w419:bool)
            n290 = Boolean To (0,1)(Boolean=w419) -> (0, 1=→"<5?":i16)
            n291 = case shown="True" w419 {
              tunnel: w427 -> [_ w441]
              frame False {
              }
              frame True {
                # "Compact\nVersion"
                n292 = local read "Past array Width"() -> (w440:dbl[])
                n293 = call "PixyAverageY.vi"("Input"=w441, "Past array Width"=w440) -> ("Array"=w439:dbl[], "mean"=w442:dbl)  [unwired: 8 in]
                n294 = local write "Past array Width"(w439) -> ()
                n295 = global write "Robot Global Data.vi" "Object Width"(w442) -> ()
              }
            }
          }
          frame True {
            w484 = 0.0 ("Height")
            # "Keep Previous value when object is lost"
            # "Zero Variables"
            n296 = local read "Lcal Pixy Out"() -> (w486:dbl)
            n297 = global write "Robot Global Data.vi" "NumValuesInTable"(w484) -> ()
          }
        }
        "Image Width" <- w408
        n298 = And(x=w417, y=w412) -> (x .and. y?=w416:bool)
        n299 = global write "Robot Global Data.vi" "Object"(w416) -> ()
        n300 = global read "Robot Global Data.vi" "Object Width"() -> (→"Averaged Values")
        n301 = local write "Lcal Pixy Out"(w409) -> ()
        n302 = global write "Robot Global Data.vi" "Object X"(w409) -> ()
        n303 = Select(t=0.0, s=w411, f=w409) -> (s? t:f=w410:dbl)
        n304 = global write "Robot Global Data.vi" "Pixy Output"(w410) -> ()
      }
      frame Enabled {
        # "Pixy Code V2\n      More Organized than V1\nShould have the same functionality as V1 which is in this structure"
        n305 = call "Pixy Logic Core.vi"() -> ()  [unwired: 12 in]
      }
    }
  }
  n306 = while {
    stop <- FALSE stop-if-true
    # "Counterpart in Shooting vi"
    # "Used to keep shoot wheel\nfrom slowing down when\na ball is shot"
    # "Shooting Ball Detection"
    n307 = call-poly <vilib>:"NT Read Value.vi"("Name"="DB/Shooting Config") -> ("Numeric Array"=w495:dbl[])  [unwired: 9 in, 1 out]
    n308 = Index Array(array=w495, index=4) -> (element=w488:dbl)
    n309 = call <vilib>:"WPI_SwitchRefNum Registry Get.vi"("refnum name"="Ball In Shooter") -> ("error out"=w492:errorcluster, "SwitchDevRef"=w491:T5)  [unwired: 9 in]
    n310 = call <vilib>:"WPI_SwitchGetLimitValue.vi"("error in (no error)"=w492, "SwitchDevRef"=w491) -> ("Switch Pressed"=w487:bool)  [unwired: 7 in, 2 out]
    n311 = global read "Robot Global Data.vi" "Shoot Latch"() -> (w497:bool)
    n312 = Equal To 0?(x=w488) -> (x = 0?=w489:bool)
    n313 = case shown="True" w489 {
      tunnel: w487 -> [w504 w506]
      tunnel: [w503 w505] -> w490
      tunnel: w488 -> [w502 _]
      frame False {
        n314 = call "Elapsed Time12"("Time Target (s)"=w502, "Reset"=w504, "Auto Reset"=w504) -> ("Time has Elapsed"=w503:bool)  [unwired: 9 in, 7 out]
      }
      frame True {
        n315 = Not(x=w506) -> (.not. x?=w505:bool)
      }
    }
    n316 = Select(t="Ball Detection Fast Time (ms)", s=w497, f=u32 100) -> (s? t:f=w499:u32)
    n317 = Wait (ms)(milliseconds to wait=w499) -> ()  [unwired: 1 out]
    n318 = case shown="True" w490 {
      frame False {
      }
      frame True {
        n319 = global write "Robot Global Data.vi" "Ball In Shooter"(TRUE) -> ()
      }
    }
  }
